vi "Tabulate_FFID_Bkgnd_Volts.vi"() -> ()   [LabVIEW 2010]
uses:
  Controls/File_Selector_Type.ctl
  Controls/Save_Data.ctl
  Controls/Setup.ctl
  Controls/Post_Process.ctl
  Globals/Meas_global.vi
panel:
  in  "At Dialog Prompt Post Process":T1=enum."Files containing the search string in the selected folder"
  in  "Search String":string="FF_Bkgnd_"
  out "current index":i32
  out "No Of files":i32
  in  "Raw Data folder":path
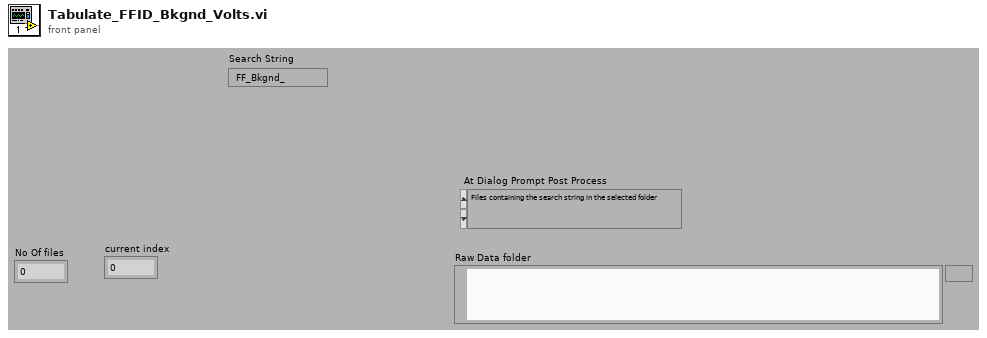
[diagram p1: front panel]
types:
  T1 = typedef "File_Selector_Type.ctl" = enum16{"The Selected File", "The Selected Folder", "Files containing the search string in the selected folder", "All files listed in selected file"}
  T2 = typedef "Save_Data.ctl" = enum16{"Save No Data", "Save Data"}
  T3 = typedef "Setup.ctl" = enum16{"Run Program", "Show Setup", "Save Current Setup", "Setup Front Panel"}
  T4 = typedef "Post_Process.ctl" = enum16{"Take New Data", "Post Process Raw Data File"}
  T5 = typedef "Analysis_info_cluster.ctl" = cluster{"Colour":u32, "Inst type":T6, "Inst name":string, "Symbol":string, "Code name":string, "Extra Info":string, "Inst Array":T7, "Index":i32, "Voltage Index":i32, "Extra Titles":string[], "Extra Values":string[]}
  T6 = typedef "Inst_type.ctl" = enum16{"Propeller anemometer", "Raw voltage", "Pressure Transducer", "Pitot-static tube", "Preston tube", "Hot wire", "Cross wire 1", "Cross wire 2", "Generic Linear", "Generic Polynomial", "Generic BackPoly", "Fast FID", "Thermocouple", "Cold wire", "Pulsed Wire", "LDA Vel", "LDA Tran time", "LDA Arr time"}
  T7 = typedef "Instrument_Array.ctl" = enum16{"PWA", "LDA", "Analogue"}
  T8 = typedef "Velocity_cluster.ctl" = cluster{"Name":string, "U":dbl, "u^2":dbl, "u^3/(u^2)^(1.5)":dbl, "u^4/(u^2)^2 -3":dbl, "% u'/U":dbl, "Mean % Err":dbl, "u^4":dbl}
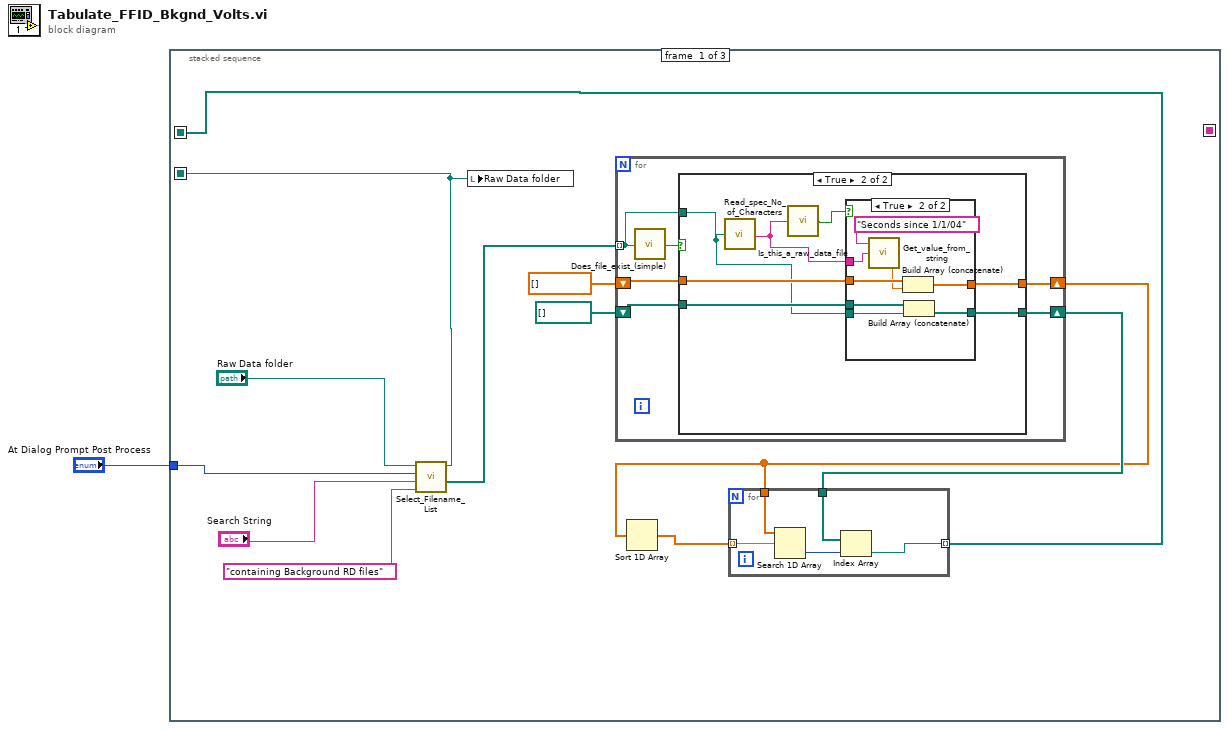
[diagram p0: block diagram]
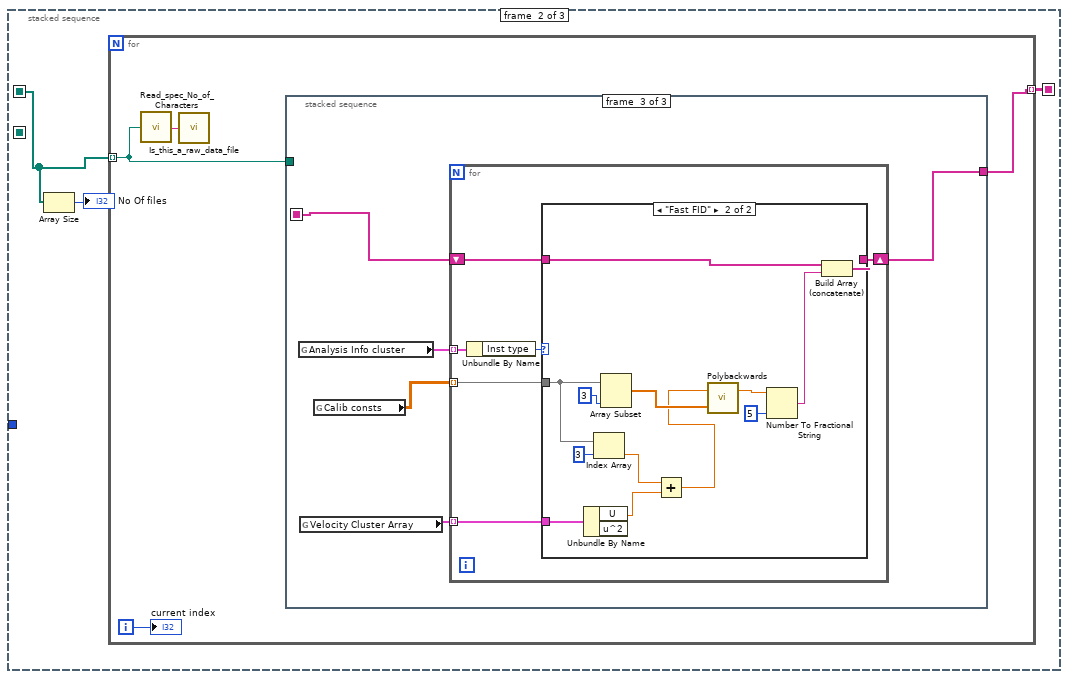
[diagram p4: hidden frame]
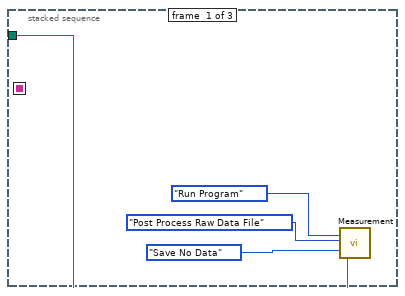
[diagram p5: hidden frame]
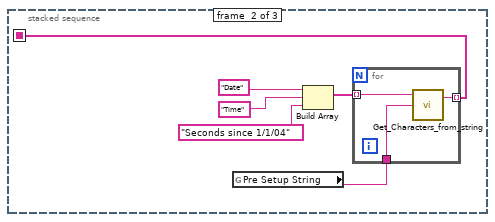
[diagram p6: hidden frame]
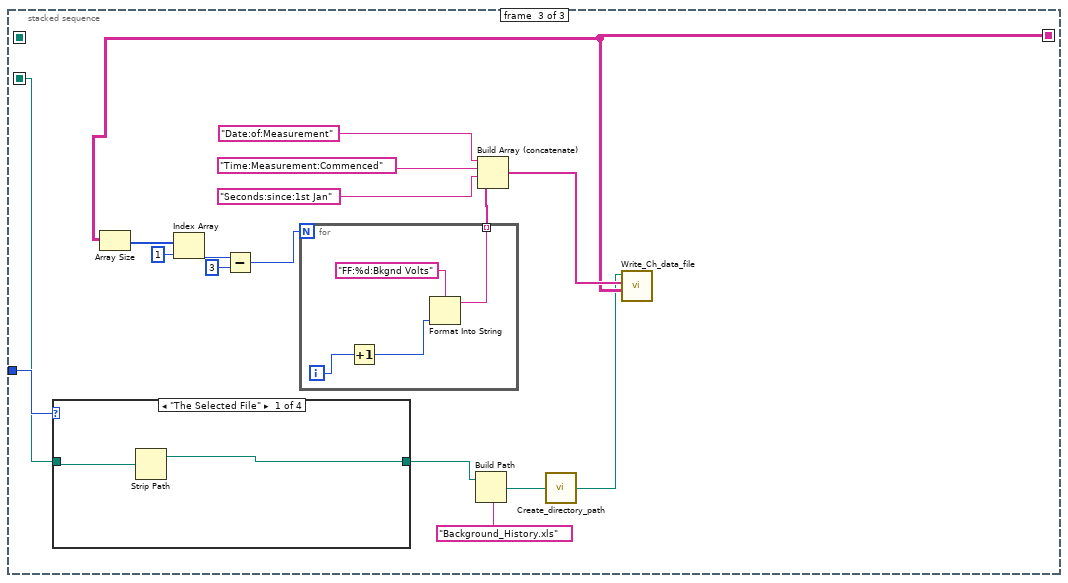
[diagram p8: hidden frame]
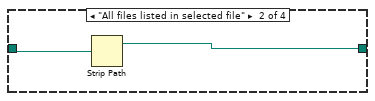
[diagram p9: hidden frame]
diagram:
  n1 = stacked-sequence {
    seq-local: [_ w44 _] -> [_ _ w95]
    seq-local: [w10 _ _] -> [_ _ w89]
    seq-local: [w3 _ _] -> [_ w45 _]
    tunnel: "At Dialog Prompt Post Process" -> [w2 _ w91]
    frame #0 {
      n2 = call "Select_Filename_List.vi"("File Type"="containing Background RD files", "Search String"="Search String", "At Dialog Prompt Post Process"=w2, "Previous Choice"="Raw Data folder") -> ("Selected files"=w4:path[], "Choosen path"=w10:path)  [unwired: 1 in, 2 out]
      n3 = local write "Raw Data folder"(w10) -> ()
      n4 = for {
        tunnel: w4 -> [w19] mode=indexing
        shift-right: [w23] -> w5
        shift-left: dbl[] [] -> [w24]
        shift-right: [w21] -> w8
        shift-left: path[] [] -> [w22]
        n5 = call "Does_file_exist_(simple).vi"("Pathname"=w19) -> ("exists?"=w20:bool)
        n6 = case shown="True" w20 {
          tunnel: w24 -> [w26 w33]
          tunnel: [w26 w32] -> w23
          tunnel: w22 -> [w25 w31]
          tunnel: [w25 w30] -> w21
          tunnel: w19 -> [_ w28]
          frame False {
          }
          frame True {
            n7 = call "Read_spec_No_of_Characters.vi"("Filename"=w28) -> ("character string"=w27:string)  [unwired: 1 out]
            n8 = call "Is_this_a_raw_data_file.vi"("character string"=w27) -> ("Raw Dat File?"=w29:bool)  [unwired: 2 out]
            n9 = case shown="True" w29 {
              tunnel: w33 -> [w35 w41]
              tunnel: [w35 w43] -> w32
              tunnel: w31 -> [w34 w39]
              tunnel: w28 -> [_ w38]
              tunnel: [w34 w37] -> w30
              tunnel: w27 -> [_ w36]
              frame False {
              }
              frame True {
                n10 = call "Get_value_from_string.vi"("Input string"=w36, "Variable name"="Seconds since 1/1/04") -> ("Value"=w40:dbl)  [unwired: 1 in, 1 out]
                n11 = Build Array (concatenate)(w41, w40) -> (w43:dbl[])
                n12 = Build Array (concatenate)(w39, w38) -> (w37:path[])
              }
            }
          }
        }
      }
      n13 = Sort 1D Array(array=w5) -> (sorted array=w6:dbl[])
      n14 = for {
        tunnel: w5 -> [w18]
        tunnel: w6 -> [w17] mode=indexing
        tunnel: w8 -> [w16]
        tunnel: [w15] -> w3 mode=indexing
        n15 = Search 1D Array(1D array=w18, element=w17) -> (index of element=w14:i32)  [unwired: 1 out]
        n16 = Index Array(array=w16, index=w14) -> (element=w15:path)
      }
    }
    frame #1 {
      n17 = Array Size(array=w45) -> (size(s)=→"No Of files":i32)
      n18 = for {
        tunnel: w45 -> [w50] mode=indexing
        tunnel: [w47] -> w44 mode=indexing
        i -> [w48]
        n19 = call "Read_spec_No_of_Characters.vi"("Filename"=w50) -> ("character string"=w49:string)  [unwired: 1 out]
        n20 = call "Is_this_a_raw_data_file.vi"("character string"=w49) -> ()  [unwired: 3 out]
        n21 = stacked-sequence {
          seq-local: [_ w55 _] -> [_ _ w65]
          tunnel: w50 -> [w51 _ _]
          tunnel: [_ _ w64] -> w47
          frame #0 {
            n22 = call "Measurement.vi"("setup"=Setup."Run Program", "Post Process"=Post_Process."Post Process Raw Data File", "File"=Save_Data."Save No Data", "Raw data file"=w51) -> ()  [unwired: 3 in, 13 out]
          }
          frame #1 {
            n23 = global read "Meas_global.vi" "Pre Setup String"() -> (w56:string)
            n24 = Build Array("Date", "Time", "Seconds since 1/1/04") -> (w57:string[])
            n25 = for {
              tunnel: w57 -> [w63] mode=indexing
              tunnel: w56 -> [w62]
              tunnel: [w61] -> w55 mode=indexing
              n26 = call "Get_Characters_from_string.vi"("Input string"=w62, "Variable name"=w63) -> ("Value"=w61:string)  [unwired: 1 in, 1 out]
            }
          }
          frame #2 {
            n27 = global read "Meas_global.vi" "Analysis Info cluster"() -> (w68:T5[])
            n28 = global read "Meas_global.vi" "Velocity Cluster Array"() -> (w66:T8[])
            n29 = global read "Meas_global.vi" "Calib consts"() -> (w67:dbl[][])
            n30 = for {
              tunnel: w68 -> [w74] mode=indexing
              tunnel: w67 -> [w73] mode=indexing
              tunnel: w66 -> [w71] mode=indexing
              shift-right: [w69] -> w64
              shift-left: w65 -> [w70]
              n31 = Unbundle By Name(w74) -> ("Inst type"=w72:T6)
              n32 = case shown="\"Fast FID\"" w72 {
                tunnel: w73 -> [_ w83]
                tunnel: w71 -> [_ w82]
                tunnel: w70 -> [w75 w79]
                tunnel: [w75 w76] -> w69
                frame "Propeller anemometer", Default {
                }
                frame "Fast FID" {
                  n33 = Unbundle By Name(w82) -> ("U"=w85:dbl)  [unwired: 1 out]
                  n34 = Index Array(array=w83, index=3 ("Index")) -> (element=w84:dbl)
                  n35 = Array Subset(array=w83, length=3 ("index")) -> (w88:dbl[])  [unwired: 1 in]
                  n36 = Add(x=w84, y=w85) -> (x+y=w81:dbl)
                  n37 = call "Polybackwards.vi"("Coefficients"=w88, "Y input"=w81) -> ("X output"=w77:dbl)  [unwired: 1 out]
                  n38 = Number To Fractional String(number=w77, precision (6)=i16 5) -> (F-format string=w78:string)  [unwired: 2 out]
                  n39 = Build Array (concatenate)(w79, w78) -> (w76:string[])
                }
              }
            }
          }
        }
        "current index" <- w48
      }
    }
    frame #2 {
      n40 = case shown="\"The Selected File\"" w91 {
        tunnel: [w106 w108 w110 w111] -> w90
        tunnel: w89 -> [w107 w109 w110 w111]
        frame "The Selected File" {
          n41 = Strip Path(path=w107) -> (stripped path=w106:path)  [unwired: 1 out]
        }
        frame "All files listed in selected file" {
          n42 = Strip Path(path=w109) -> (stripped path=w108:path)  [unwired: 1 out]
        }
        frame "Files containing the search string in the selected folder" {
        }
        frame "The Selected Folder" {
        }
      }
      n43 = Array Size(array=w95) -> (size(s)=w105:i32[])
      n44 = Index Array(array=w105, index=1) -> (element=w96:i32)
      n45 = Subtract(x=w96, y=3) -> (x-y=w102:i32)
      n46 = for {
        N: w102 -> [_]
        tunnel: [w112] -> w98 mode=indexing
        i -> [w115]
        n47 = Increment(x=w115) -> (x+1=w114:i32)
        n48 = Format Into String(format string="FF:%d:Bkgnd Volts", w114) -> (resulting string=w112:string)  [unwired: 2 in, 1 out]
      }
      n49 = Build Path(base path=w90, name or relative path="Background_History.xls") -> (appended path=w93:path)
      n50 = Build Array (concatenate)("Date:of:Measurement", "Time:Measurement:Commenced", "Seconds:since:1st Jan", w98) -> (w97:string[])
      n51 = call "Create_directory_path.vi"("Path name"=w93) -> ("Path name Out"=w92:path)
      n52 = call "Write_Ch_data_file.vi"("Channel Values"=w95, "Channel names"=w97, "Filename"=w92) -> ()  [unwired: 5 in, 4 out]
    }
  }
